vi "Update I2C Monitor Table.vi"(6 "Transactions Limit (10k)":i32=10000 format="%.0p", 7 "# TXNS IN TABLE Ref":refnum<vi>, 8 "error in (no error)":errorcluster, 10 "I2C Data in":string[][](array[string]), 11 "I2C Table Ref":refnum<vi>) -> (0 "error out":errorcluster)   [LabVIEW 2025, in "I2C Bus Monitor UI.lvlib"]
uses:
  I2C Bus Monitor UI.lvlib
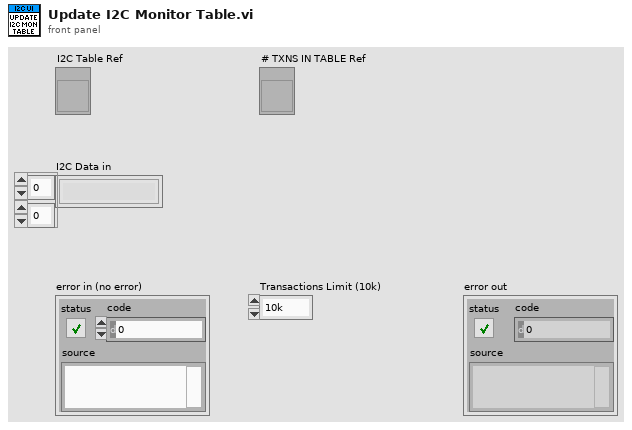
[diagram p1: front panel]
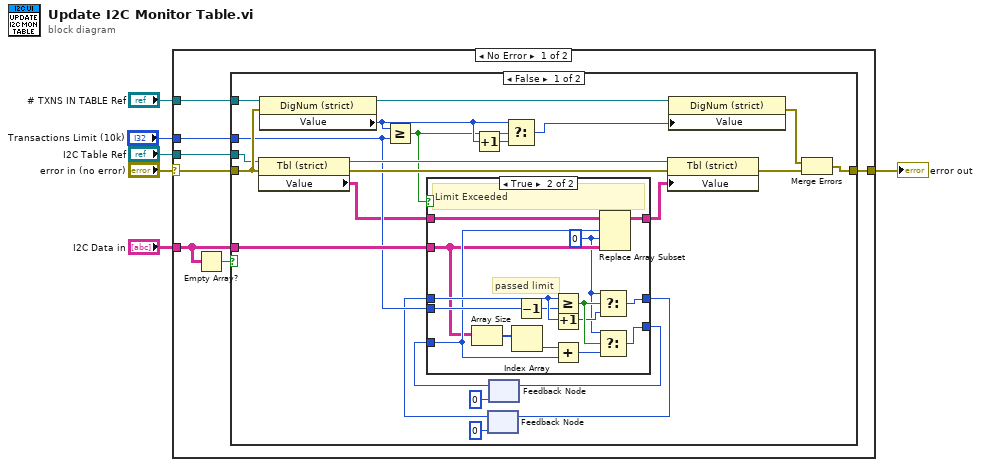
[diagram p0: block diagram]
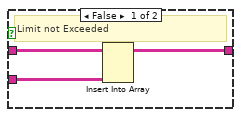
[diagram p2: hidden frame]
diagram:
  n1 = case shown="No Error" "error in (no error)" {
    selector: "error in (no error)" -> [w12 w56]
    tunnel: "I2C Table Ref" -> [w13 _]
    tunnel: "I2C Data in" -> [w9 _]
    tunnel: [w11 w56] -> w3
    tunnel: "# TXNS IN TABLE Ref" -> [w8 _]
    tunnel: "Transactions Limit (10k)" -> [w7 _]
    frame No Error {
      n2 = Empty Array?(array=w9) -> (empty?=w10:bool)
      n3 = case shown="False" w10 {
        tunnel: w9 -> [w24 _]
        tunnel: w13 -> [w35 _]
        tunnel: w12 -> [w36 w55]
        tunnel: [w29 w55] -> w11
        tunnel: w8 -> [w31 _]
        tunnel: w7 -> [w19 _]
        frame False {
          n4 = property on="Property Node" class="Tbl (strict)"(reference=w35, error in=w36) -> (reference out=w34:refnum<vi>, error out=w32:errorcluster, "Value"=w15:string[][])
          n5 = property on="Property Node" class="DigNum (strict)"(reference=w31, error in=w36) -> (reference out=w30:refnum<vi>, "Value"=w26:i32)  [unwired: 1 out]
          n6 = Greater Or Equal?(x=w26, y=w19) -> (x >= y?=w23:bool)
          n7 = Increment(x=w26) -> (x+1=w27:i32)
          n8 = feedback #1(0 ("index (row)")) -> (w14:i32)
          n9 = feedback #2(0 ("index (row)")) -> (w21:i32)
          n10 = case shown="True" w23 {
            tunnel: w15 -> [w39 w54]
            tunnel: [w38 w52] -> w18
            tunnel: w24 -> [w37 w43]
            tunnel: w21 -> [_ w44]
            tunnel: [_ w50] -> w22
            tunnel: w19 -> [_ w49]
            tunnel: [_ w47] -> w16
            tunnel: w14 -> [_ w46]
            frame False {
              # "Limit not Exceeded"
              n11 = Insert Into Array(array=w39, new element=w37) -> (w38:string[][])  [unwired: 2 in]
            }
            frame True {
              w40 = 0 ("disabled index (col)")
              # "passed limit"
              # "Limit Exceeded"
              n12 = Array Size(array=w43) -> (size(s)=w53:i32[])
              n13 = Index Array(array=w53) -> (element=w42:i32)  [unwired: 1 in]
              n14 = Decrement(x=w49) -> (x-1=w41:i32)
              n15 = Greater Or Equal?(x=w46, y=w41) -> (x >= y?=w48:bool)
              n16 = Increment(x=w46) -> (x+1=w45:i32)
              n17 = Add(x=w42, y=w44) -> (x+y=w51:i32)
              n18 = Select(t=w40, s=w48, f=w45) -> (s? t:f=w47:i32)
              n19 = Select(t=w40, s=w48, f=w51) -> (s? t:f=w50:i32)
              n20 = Replace Array Subset(array=w54, new element=w43, index (row)=w44, index (col)=w40) -> (w52:string[][])
            }
          }
          n21 = feedback-in #1(w16) -> ()
          n22 = feedback-in #2(w22) -> ()
          n23 = Select(t=w26, s=w23, f=w27) -> (s? t:f=w25:i32)
          n24 = property on="Property Node" class="Tbl (strict)"(reference=w34, error in=w32, "Value"=w18) -> (error out=w33:errorcluster)  [unwired: 1 out]
          n25 = property on="Property Node" class="DigNum (strict)"(reference=w30, "Value"=w25) -> (error out=w28:errorcluster)  [unwired: 1 in, 1 out]
          n26 = Merge Errors(w28, w33) -> (w29:errorcluster)
        }
        frame True {
        }
      }
    }
    frame Error {
    }
  }
  "error out" <- w3
